vi "asdf.vi"(8 "error in":errorcluster {"code" min=0 max=0}, 11 "Icon data":T1={"Text Visible?"=FALSE, "Text Opacity"=0, "Templ Visible?"=FALSE, "Templ Opacity"=0, "Relative Path from 1 to 2"=path "", "Image"=bytes[0], "All User Layers"=[], "Body Text"={"Line 1 text"="", "Line 2 text"="", "Line 3 text"="", "Line 4 text"="", "Line 1 color"=0, "Line 2 color"=0, "Line 3 color"=0, "Line 4 color"=0, "Body Text Spec"={"Font"="", "Alignment"=0, "Size"=3}, "Center text vertically"=FALSE, "Capitalize Text"=FALSE}} {"Body Text"."Body Text Spec"."Alignment" items=["left", "center", "right"]}) -> (0 "error out":errorcluster {"code" min=0 max=0}, 3 "data string":string)   [LabVIEW 2018]
uses:
  <vilib>/LabVIEW Icon API/lv_icon/Classes/Load_Unload/Load & Unload.lvclass
  <vilib>/LabVIEW Icon API/lv_icon/lv_icon.lvlib
  <vilib>/LabVIEW Icon API/lv_icon/Classes/Layer/Layer.lvclass
  <vilib>/LabVIEW Icon API/lv_icon/Controls/Font.ctl
  <vilib>/LabVIEW Icon API/lv_icon/Controls/BodyText.ctl
  <vilib>/LabVIEW Icon API/lv_icon/Controls/Alignment.ctl
  <vilib>/LabVIEW Icon API/lv_icon/Controls/LabVIEW Icon Stored Information.ctl
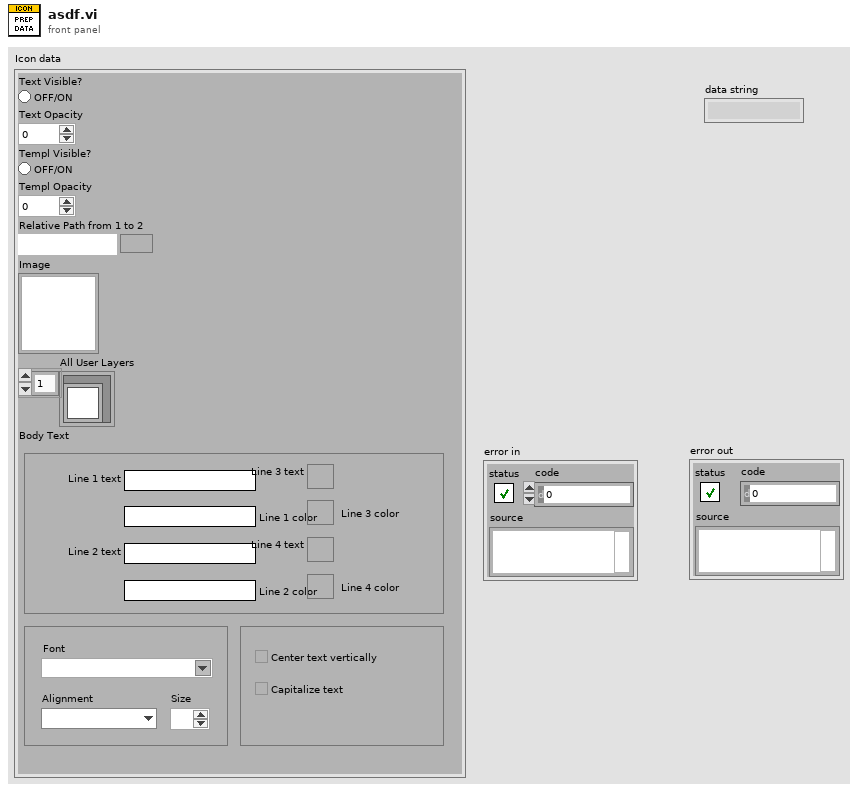
[diagram p1: front panel]
types:
  T1 = typedef "LabVIEW Icon Stored Information.ctl" = cluster{"Text Visible?":bool, "Text Opacity":u8, "Templ Visible?":bool, "Templ Opacity":u8, "Relative Path from 1 to 2":path, "Image":picture, "All User Layers":refnum<class "Layer.lvclass">[], "Body Text":T2}
  T2 = typedef "BodyText.ctl" = cluster{"Line 1 text":string, "Line 2 text":string, "Line 3 text":string, "Line 4 text":string, "Line 1 color":u32, "Line 2 color":u32, "Line 3 color":u32, "Line 4 color":u32, "Body Text Spec":cluster{"Font":T3, "Alignment":T4, "Size":u8}, "Center text vertically":bool, "Capitalize Text":bool}
  T3 = typedef "Font.ctl" = string
  T4 = typedef "Alignment.ctl" = u16
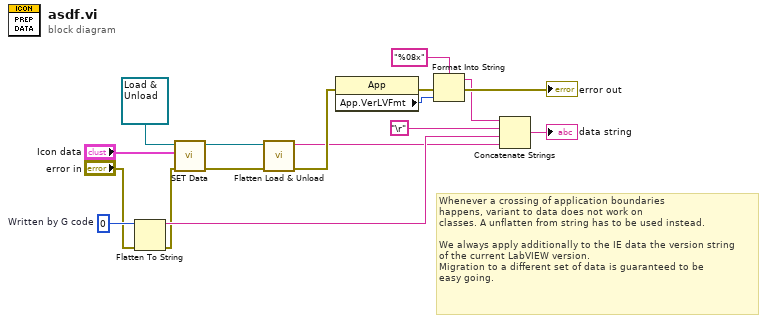
[diagram p0: block diagram]
diagram:
  w8 = u8 0  # Written by G code
  # "Whenever a crossing of application boundaries\nhappens, variant to data does not work on \nclasses. A unflatten from string has to be used instead.\n\nWe always apply additionally to the IE data the version string\nof the current LabVIEW version.\nMigration to a different set of data is guaranteed to be\neasy going."
  n1 = Flatten To String(anything=w8, error in (no error)="error in") -> (data string=w7:string, error out=w5:errorcluster)  [unwired: 2 in, 1 out]
  n2 = call-dynamic "SET Data.vi"("error in (no error)"=w5, "Data"="Icon data", "Load & Unload.lvclass in"=refnum<class "Load & Unload.lvclass"> refnum) -> ("error out"=w4:errorcluster, "Load & Unload.lvclass out"=w1:refnum<class "Load & Unload.lvclass">)  [unwired: 7 in]
  n3 = call <vilib>:"Flatten Load & Unload.vi"("Error In"=w4, "Load & Unload.lvclass"=w1) -> ("Error Out"=w3:errorcluster, "String"=w2:string)  [unwired: 8 in]
  n4 = property class="App"(error in=w3) -> (error out=w13:errorcluster, "App.VerLVFmt"=w11:i32)  [unwired: 1 in, 1 out]
  n5 = Format Into String(format string="%08x", error in=w13, w11) -> (resulting string=w9:string, error out=→"error out":errorcluster)  [unwired: 1 in]
  n6 = Concatenate Strings(w9, "\r", w7, w2) -> (→"data string":string)
